vi "Compute Optimal IRF v4.vi"(6 "Laser Period":dbl[unit], 7 "Decay Fit Options":T1={"Show Fit Residuals"=TRUE, "Fit Model"=enum."1-Exponential", "Residual Type"=enum."Standard", "Max Decay Percentile"=0.0, "Min Decay Percentile"=0.0, "Show Full Decay"=TRUE, "Weights"=enum."Unweighted", "Fitting Method"=enum."Least Square", "Compute Parameter Uncertainties"=TRUE, "Periodic Boundaries"=TRUE, "Model Calculation"=enum."Simulation", "Period"=1.2500000000000001e-08, "Termination Criteria"={"Max Iterations"=0, "Max Function Calls"=0, "Max Time"=1000.0, "Function Tolerance"=1e-06, "Parameter Tolerance"=1e-06, "Gradient Tolerance"=0.0, "Min Lambda"=1e-06, "Max Lambda"=1e-06, "Initial Tick Count"=0}, "Offset Resolution"=1.2500000000000001e-08, "Use Local IRF"=TRUE, "Fitting Algorithm"=enum."Levenberg-Marquardt", "Show Confidence Interval "=TRUE, "Confidence Level"=95.0} {"Confidence Level" min=0.0 max=100.0; "Offset Resolution" min=0.0; "Period" min=0.0; "Min Decay Percentile" min=0.0 max=1.0; "Max Decay Percentile" min=0.0 max=100.0}, 8 "Error In":errorcluster, 9 "IRF Optimization Control":T12={"Search Range"=1e-18, "Search Step"=1e-18, "Tail Threshold (%)"=1e-09, "Regularized IRF"=FALSE, "Export Plot"=FALSE, "Export Data"=FALSE, "Smooth Metrics"=FALSE, "S-G Side Points"=1, "S-G Polynomial Order"=3, "Metrics"=enum."Tail Average"} {"S-G Polynomial Order" min=3 max=10; "S-G Side Points" min=1; "Tail Threshold (%)" min=0.0 max=100.0; "Search Range" min=0.0 max=1e-09}, 10 "Extract IRF Options":T8={"Time Constant for IRF Extraction"=1e-18, "IRF Order"=1, "Fourier Series Smoothing"=enum."None", "Noise Threshold"=0.0, "Smoothing Width"=0.0, "Fourier Series Truncation"=enum."Automatic", "Truncation Order"=0, "Save Power Spectrum"=FALSE, "Smoothing"=FALSE, "Smoothing Parameter"=0.0, "Smoothing Order"=1, "Method"=enum."Direct"} {"Smoothing Order" min=1 max=10; "Time Constant for IRF Extraction" format="%#_5g"}, 11 "Selected Plot Info":T14={"Multiplot XY Graph"=refnum, "Mouse Coordinates"={"Horizontal"=0, "Vertical"=0}, "Plot Index"=-1}) -> (0 "Error Out":errorcluster, 1 "Optimal Tau":dbl, 2 "Plot Name":string, 3 "IRF Plot":cluster{"X Array":dbl[], "Y Array":dbl[]}, 4 "Optimal IRF Results String":string, 5 "Optimization Graph":cluster{dbl[], dbl[]}[](graph))   [LabVIEW 2021, in "AlliGator IRF.lvlib"]
doc: "Extract IRF from provided decay and time constant"
uses:
  AlliGator/Decay Analysis/IRF/AlliGator IRF.lvlib
  Graphs/XY Graph/XY Graph Selected Plot Info.ctl
  Graphs/XY Graph/XY Graph Refnum.ctl
  <vilib>/Utility/miscctls.llb/LVPoint32TypeDef.ctl
  AlliGator/Decay Analysis/IRF/AlliGator IRF Optimization Controls.ctl
  AlliGator/Decay Analysis/IRF/AlliGator IRF Deconvolution Metrics.ctl
  IRF(X)PSED Extraction Options.ctl
  Fourier Series Smoothing Option.ctl
  Fourier Series Truncation.ctl
  IRF Extraction Method.ctl
  Decay Fit Options v4.ctl
  Decay Convolution/Decay Model.ctl
  Residual Type.ctl
  Fit Weights Type v2.ctl
  Non-linear Fitting Method v2.ctl
  Fit Calculation Method.ctl
  Non-linear Fitting Algorithm.ctl
  Fit Plot Request Information.ctl
  <vilib>/Utility/miscctls.llb/LVPointDoubleTypeDef.ctl
  Fit Models.ctl
  cc3fc4cb-3fe6-4f43-9f61-aa3a5ef9d036.vi
  <vilib>/Analysis/1siggen.llb/Ramp Pattern by Delta.vi
  Decay Convolution/LM model function and gradient (1-Exp, Convolved, Periodic, Fixed Parameters) v3.vi
  <userlib>/_OpenG.lib/array/array.llb/Filter 1D Array with Scalar (DBL)__ogtk.vi
  <userlib>/_OpenG.lib/array/array.llb/Delete Elements from 1D Array (DBL)__ogtk.vi
  <vilib>/Analysis/NI_AALBase.lvlib
  Time/Time.lvlib
  Fits.lvlib
  Utilities/Utilities.lvlib
  Arrays/Arrays.lvlib
  Graphs/XY Graph/XY Graph Add-Ons.lvlib
  <vilib>/Analysis/NI_AALPro.lvlib
  <userlib>/_OpenG.lib/array/array.llb/openg_array.lvlib
  AlliGator/Decay Analysis/Decay Fit/AlliGator Decay Fit.lvlib
panel:
  in  "Display":bool
  out "# Tail Points":i32
  out "min value":dbl
  in  "Debug":bool
  out "IRF Graph":cluster{"X Array":dbl[], "Y Array":dbl[]}[](graph)
  out "Current Tau (ns)":dbl format="%#_4g"
  # "1. In debug mode, move the cursor in the Optimization Graph to display the corresponding IRF in the IRF Graph\n2. Click on the close window X to stop debugging"
  # "see the AlliGator License on the block diagram (Ctrl+E or Window:Show Block Diagram)"
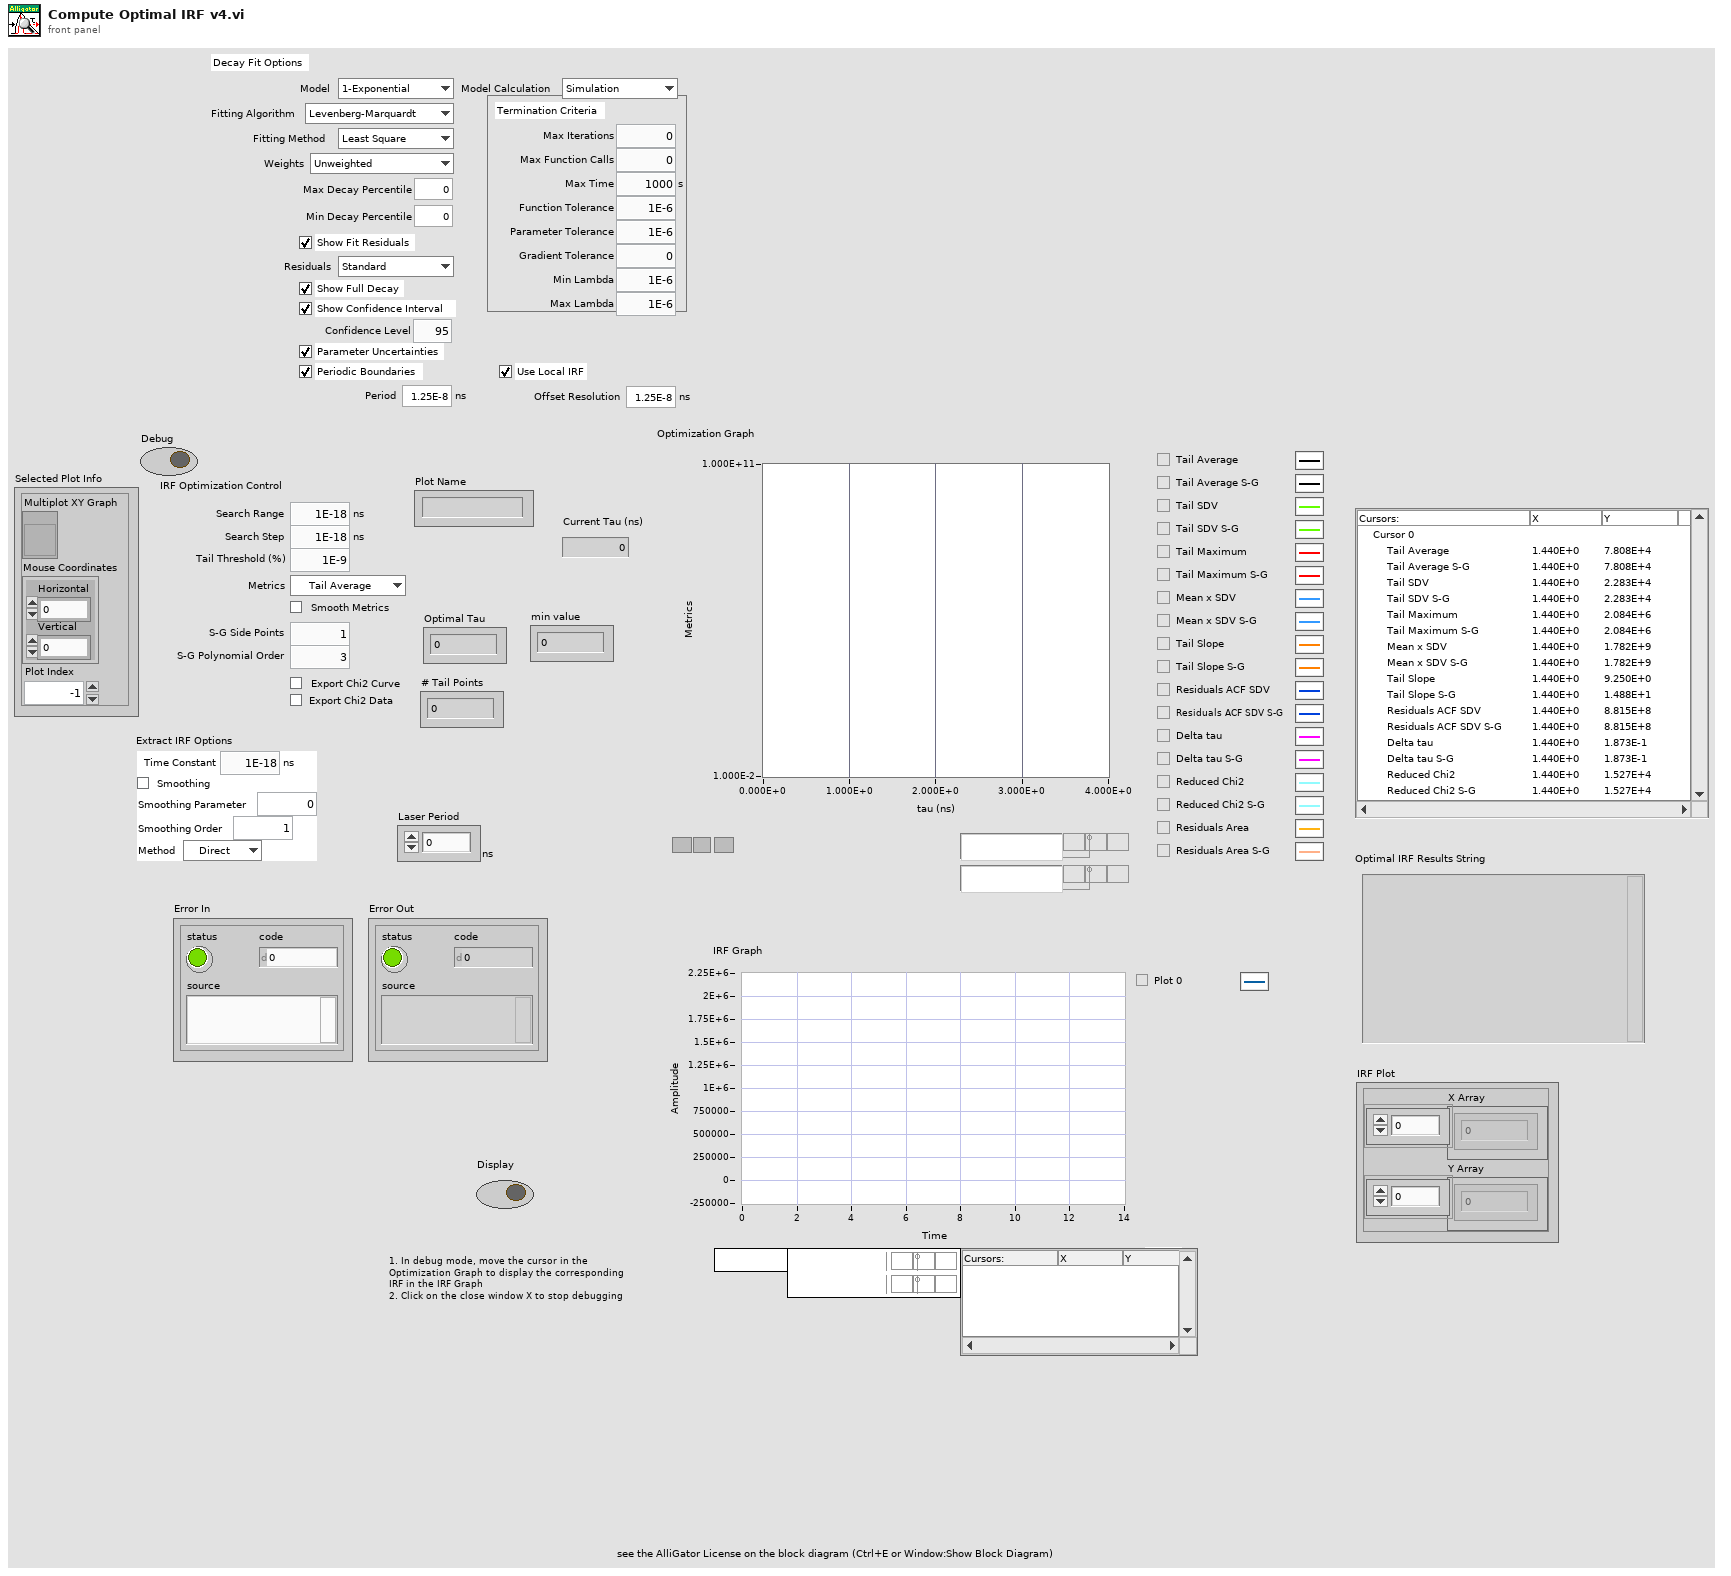
[diagram p1: front panel]
types:
  T1 = typedef "Fits.lvlib/Decay Fit Options v4.ctl" = cluster{"Show Fit Residuals":bool, "Fit Model":T2, "Residual Type":T3, "Max Decay Percentile":dbl, "Min Decay Percentile":dbl, "Show Full Decay":bool, "Weights":T4, "Fitting Method":T5, "Compute Parameter Uncertainties":bool, "Periodic Boundaries":bool, "Model Calculation":T6, "Period":dbl[unit], "Termination Criteria":cluster{"Max Iterations":i32, "Max Function Calls":i32, "Max Time":dbl[unit], "Function Tolerance":dbl, "Parameter Tolerance":dbl, "Gradient Tolerance":dbl, "Min Lambda":dbl, "Max Lambda":dbl, "Initial Tick Count":u32}, "Offset Resolution":dbl[unit], "Use Local IRF":bool, "Fitting Algorithm":T7, "Show Confidence Interval ":bool, "Confidence Level":dbl}
  T2 = typedef "Fits.lvlib/Decay Model.ctl" = enum16{"1-Exponential", "2-Exponentials"}
  T3 = typedef "Fits.lvlib/Residual Type.ctl" = enum16{"Standard", "Normalized", "Reduced"}
  T4 = typedef "Fits.lvlib/Fit Weights Type v2.ctl" = enum16{"Unweighted", "1/Variance (Neyman)", "1/Variance (Pearson)", "Best of All"}
  T5 = typedef "Fits.lvlib/Non-linear Fitting Method v2.ctl" = enum16{"Least Square", "Least Absolute Residual", "Bisquare", "MLE", "-", "Best of All"}
  T6 = typedef "Fits.lvlib/Fit Calculation Method.ctl" = enum16{"Simulation", "Convolution", "Integration"}
  T7 = typedef "Fits.lvlib/Non-linear Fitting Algorithm.ctl" = enum16{"Levenberg-Marquardt", "Trust-Region Dogleg"}
  T8 = typedef "Fits.lvlib/IRF(X)PSED Extraction Options.ctl" = cluster{"Time Constant for IRF Extraction":dbl[unit], "IRF Order":i32, "Fourier Series Smoothing":T9, "Noise Threshold":dbl, "Smoothing Width":dbl, "Fourier Series Truncation":T10, "Truncation Order":i32, "Save Power Spectrum":bool, "Smoothing":bool, "Smoothing Parameter":dbl, "Smoothing Order":u32, "Method":T11}
  T9 = typedef "Fits.lvlib/Fourier Series Smoothing Option.ctl" = enum16{"None", "Lanczos Factors", "Fejer Summation"}
  T10 = typedef "Fits.lvlib/Fourier Series Truncation.ctl" = enum16{"Automatic", "Fixed"}
  T11 = typedef "Fits.lvlib/IRF Extraction Method.ctl" = enum16{"Direct", "Topless", "Toeplitz"}
  T12 = typedef "AlliGator IRF.lvlib/AlliGator IRF Optimization Controls.ctl" = cluster{"Search Range":dbl[unit], "Search Step":dbl[unit], "Tail Threshold (%)":dbl, "Regularized IRF":bool, "Export Plot":bool, "Export Data":bool, "Smooth Metrics":bool, "S-G Side Points":i32, "S-G Polynomial Order":i32, "Metrics":T13}
  T13 = typedef "AlliGator IRF.lvlib/AlliGator IRF Deconvolution Metrics.ctl" = enum16{"Tail Average", "Tail SDV", "Tail Max", "Tail Average * SDV", "Tail Slope", "Residuals ACF SDV", "Delta tau", "Reduced Chi2", "Residuals Area"}
  T14 = typedef "XY Graph Add-Ons.lvlib/XY Graph Selected Plot Info.ctl" = cluster{"Multiplot XY Graph":T15, "Mouse Coordinates":T16, "Plot Index":i32}
  T15 = typedef "XY Graph Add-Ons.lvlib/XY Graph Refnum.ctl" = refnum<vi>
  T16 = typedef "LVPoint32TypeDef.ctl" = cluster{"Horizontal":i32, "Vertical":i32}
  T17 = typedef "Fits.lvlib/Fit Plot Request Information.ctl" = cluster{"XY Graph Ref":refnum<vi>, "Mouse Coordinates":T18, "Fit Model":T19, "Plot Index":i32}
  T18 = typedef "LVPointDoubleTypeDef.ctl" = cluster{"X":dbl, "Y":dbl}
  T19 = typedef "Fits.lvlib/Fit Models.ctl" = enum16{"Select a Fit Model...", "           Single Peak", "Gaussian", "Asymmetric Gaussian", "Lorentzian", "Asymmetric Lorentzian", "Gaussian/Lorentzian", "Lorentzian/Gaussian", "           Double Peak", "Two Gaussians", "Two Asymmetric Gaussians", "Two H-Connected Gaussians", "Two T-Connected Gaussians", "Two H-Connected Asymmetric Gaussians", "Two T-Connected Asymmetric Gaussians", "           Triple Peak", "Three Gaussians", "Three Asymmetric Gaussians", "              Decays", "1-Exponential", "IRF*PSED", "2-Exponentials", "            Power Law", "Power Law", "Power Law with Offset", "               ACF", "2D Gaussian ACF", "2D Gaussian + Blinking ACF", "2D Gaussian + Flow ACF", "3D Gaussian ACF", "3D Gaussian + Blinking ACF", "             Multiplot", "2D Gaussian ACF & 2D Gaussian + Flow ACF"}
  T20 = typedef "XY Graph Add-Ons.lvlib/XY Graph Plot Data.ctl" = cluster{"X Array":dbl[], "Y Array":dbl[]}
  T21 = typedef "Fits.lvlib/Decay Fit Parameter Constraints Arrays.ctl" = cluster{"Parameter Bounds (Fix+Fit)":cluster{"parameter minimum":dbl[], "parameter maximum":dbl[]}, "Fitted Parameters":T22[], "Fixed Parameters":T22[], "Fit Model":T2}
  T22 = typedef "Fits.lvlib/Decay Fit Parameters In List.ctl" = enum16{"Offset", "Baseline", "A_1", "tau_1", "A_2", "tau_2"}
  T23 = cluster{"t Array (dup)":dbl[], "IRF Array":dbl[]}
  T24 = typedef "Fits.lvlib/Fit Plots.ctl" = cluster{"Fitted Decay":cluster{"t Array":dbl[], "Fitted Array":dbl[]}, "Residuals":cluster{"t Array":dbl[], "Residual Array":dbl[]}, "Upper CI Plot":cluster{"t Array":dbl[], "Residual Array":dbl[]}, "Lower CI Plot":cluster{"t Array":dbl[], "Residual Array":dbl[]}}
  T25 = typedef "Fits.lvlib/Non-linear Fit Output v4.ctl" = cluster{"best nonlinear fit":dbl[], "best fit parameters":dbl[], "R^2":dbl, "RMSE":dbl, "error out":errorcluster, "Fitting Method":T26, "number of function calls":i32, "number of iterations":i32, "covariance":T27, "Chi 2":dbl, "DOF":i32, "Fit Convergence Criterion":T28, "Fitting Algorithm":T7, "Weighted Fit":T4, "Gradient":dbl, "|Delta Chi 2|":dbl, "|Delta Chi 2|/Chi 2":dbl, "Max |Delta a| /|a|":dbl, "Lambda":dbl, "RSS":dbl, "AIC":dbl, "BIC":dbl, "Max number of function calls":i32, "Max number of iterations":i32, "IRF":T20, "IRF Normalization Factor":dbl, "Decay Normalization Factor":dbl, "Number of offset fits":i32, "Weighted Chi2":dbl, "Unweighted Chi2":dbl}
  T26 = typedef "Fits.lvlib/Nonlinear Fit Method.ctl" = enum16{"Least Square", "Least Absolute Residual", "Bisquare", "MLE"}
  T27 = typedef "NI_Matrix.lvlib/RealMatrix.ctl" = dbl[][]
  T28 = typedef "Fits.lvlib/Convergence Criteria.ctl" = enum16{"Continue", "Tolerances Exceeded", "Max Time Exceeded", "Max Iterations Exceeded", "Max Function Evaluations Exceeded", "Scale Range Exceeded"}
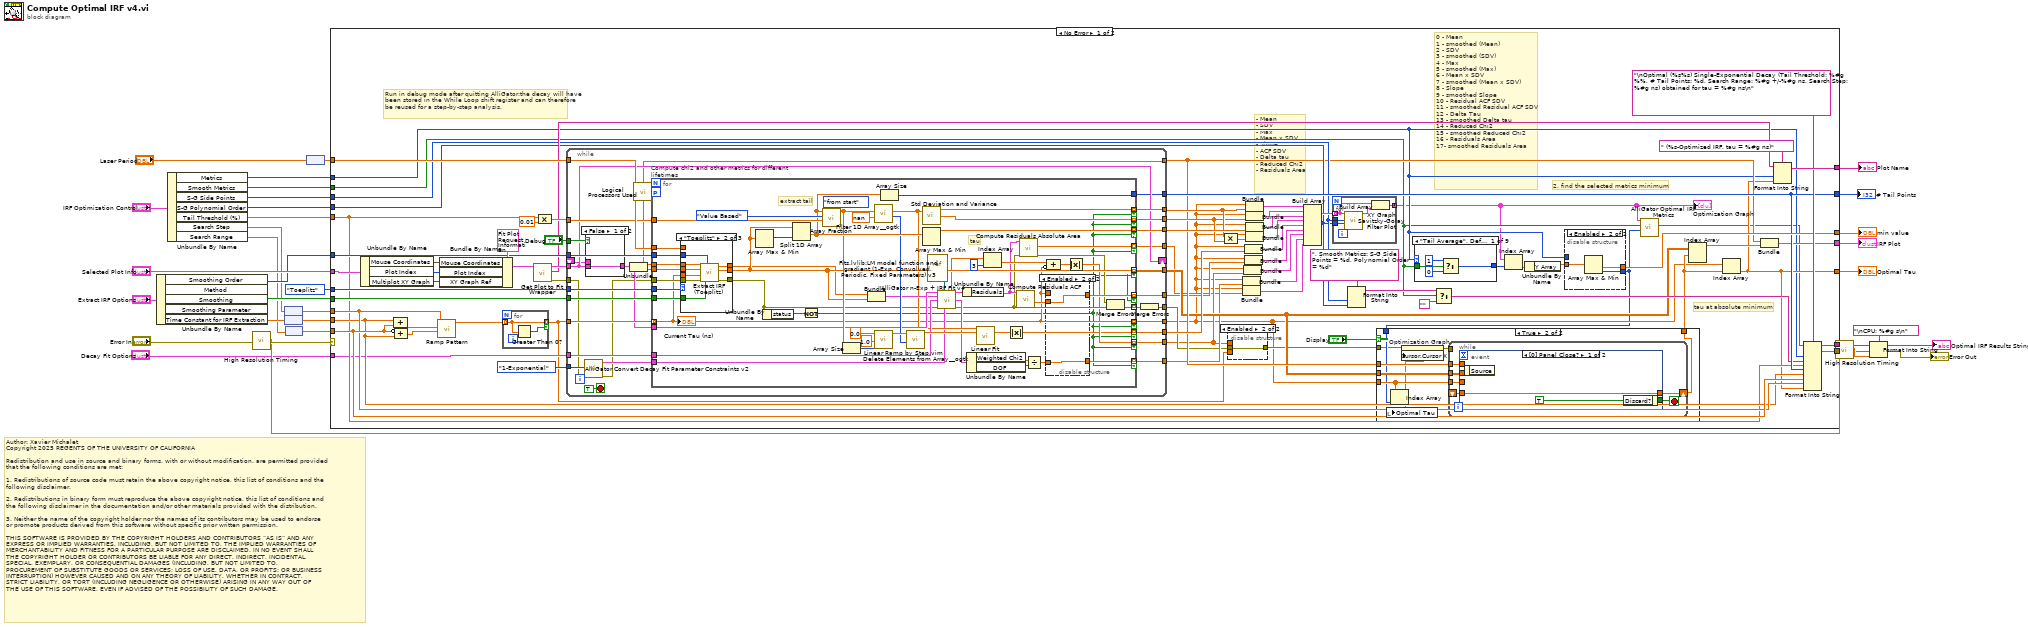
[diagram p0: block diagram]
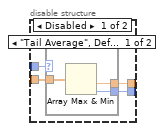
[diagram p2: hidden frame]
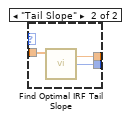
[diagram p3: hidden frame]
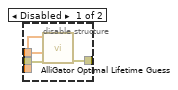
[diagram p4: hidden frame]
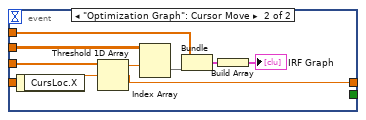
[diagram p6: hidden frame]
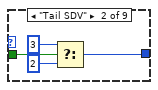
[diagram p7: hidden frame]
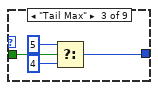
[diagram p8: hidden frame]
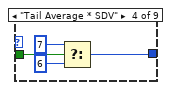
[diagram p9: hidden frame]
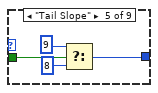
[diagram p10: hidden frame]
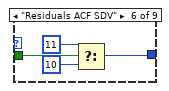
[diagram p11: hidden frame]
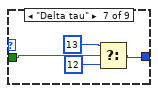
[diagram p12: hidden frame]
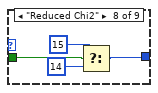
[diagram p13: hidden frame]
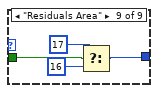
[diagram p14: hidden frame]
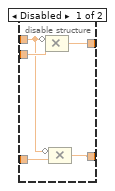
[diagram p15: hidden frame]
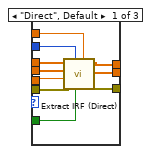
[diagram p16: hidden frame]
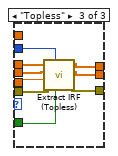
[diagram p17: hidden frame]
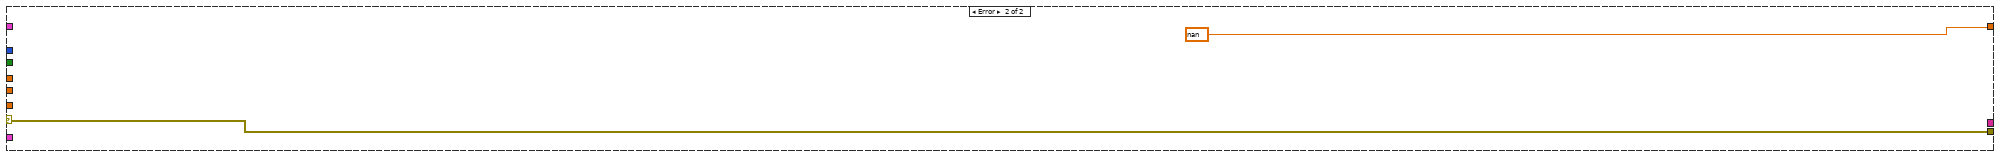
[diagram p19: hidden frame]
diagram:
  # "Author: Xavier Michalet\nCopyright 2025 REGENTS OF THE UNIVERSITY OF CALIFORNIA\n\nRedistribution and use in source and binary forms, with or without modification, are permitted provided\nthat the following conditions are met:\n\n1. Redistributions of source code must retain the above copyright notice, this list of conditions and the\nfollowing disclaimer.\n\n2. Redistributions in binary form must reproduce the above copyright notice, this list of conditions and\nthe following disclaimer in the documentation and/or other materials provided with the distribution.\n\n3. Neither the name of the copyright holder nor the names of its contributors may be used to endorse \nor promote products derived from this software without specific prior written permission.\n\nTHIS SOFTWARE IS PROVIDED BY THE COPYRIGHT HOLDERS AND CONTRIBUTORS “AS IS” AND ANY \nEXPRESS OR IMPLIED WARRANTIES, INCLUDING, BUT NOT LIMITED TO, THE IMPLIED WARRANTIES OF\nMERCHANTABILITY AND FITNESS FOR A PARTICULAR PURPOSE ARE DISCLAIMED. IN NO EVENT SHALL\nTHE COPYRIGHT HOLDER OR CONTRIBUTORS BE LIABLE FOR ANY DIRECT, INDIRECT, INCIDENTAL, \nSPECIAL, EXEMPLARY, OR CONSEQUENTIAL DAMAGES (INCLUDING, BUT NOT LIMITED TO, \nPROCUREMENT OF SUBSTITUTE GOODS OR SERVICES; LOSS OF USE, DATA, OR PROFITS; OR BUSINESS\nINTERRUPTION) HOWEVER CAUSED AND ON ANY THEORY OF LIABILITY, WHETHER IN CONTRACT, \nSTRICT LIABILITY, OR TORT (INCLUDING NEGLIGENCE OR OTHERWISE) ARISING IN ANY WAY OUT OF\nTHE USE OF THIS SOFTWARE, EVEN IF ADVISED OF THE POSSIBILITY OF SUCH DAMAGE."
  n1 = Unbundle By Name("Extract IRF Options") -> ("Smoothing Order"=w21:u32, "Smoothing"=w20:bool, "Time Constant for IRF Extraction"=w23:dbl[unit])  [unwired: 2 out]
  n2 = Unbundle By Name("IRF Optimization Control") -> ("Metrics"=w5:T13, "Smooth Metrics"=w8:bool, "S-G Side Points"=w7:i32, "S-G Polynomial Order"=w6:i32, "Tail Threshold (%)"=w15:dbl, "Search Step"=w14:dbl[unit], "Search Range"=w12:dbl[unit])
  n3 = call "High Resolution Timing.vi"("Error In"="Error In") -> ("elapsed (relative) seconds"=w30:dbl, "Error Out"=w34:errorcluster)  [unwired: 16 in, 1 out]
  n4 = node(w14) -> (w33:dbl)
  n5 = node(w23) -> (w32:dbl)
  n6 = node(w12) -> (w11:dbl)
  n7 = node("Laser Period") -> (w17:dbl)
  n8 = case shown="No Error" w34 {
    selector: w34 -> [_ w325]
    tunnel: [w94 w325] -> w35
    tunnel: w32 -> [w76 _]
    tunnel: w33 -> [w81 _]
    tunnel: w11 -> [w82 _]
    tunnel: "Selected Plot Info" -> [w109 _]
    tunnel: [w95 _] -> w29
    tunnel: [w62 _] -> w22
    tunnel: w21 -> [w102 _]
    tunnel: w20 -> [w101 _]
    tunnel: [w50 nan] -> w19
    tunnel: [w97 _] -> w18
    tunnel: w15 -> [w71 _]
    tunnel: IRF_Extraction_Method."Toeplitz" ("Method") -> [w93 _]
    tunnel: w17 -> [w92 _]
    tunnel: [w79 _] -> w10
    tunnel: [w77 _] -> w9
    tunnel: w8 -> [w39 _]
    tunnel: w7 -> [w68 _]
    tunnel: w6 -> [w67 _]
    tunnel: w5 -> [w49 _]
    tunnel: "Decay Fit Options" -> [w56 _]
    frame No Error {
      # "Run in debug mode after quitting AlliGator:the decay will have been stored in the While Loop shift register and can therefore be reused for a step-by-step analysis."
      # "0 - Mean\n1 - smoothed (Mean)\n2 - SDV\n3 - smoothed (SDV)\n4 - Max\n5 - smoothed (Max)\n6 - Mean x SDV\n7 - smoothed (Mean x SDV)\n8 - Slope\n9 - smoothed Slope\n10 - Residual ACF SDV\n11 - smoothed Residual ACF SDV\n12 - Delta Tau\n13 - smoothed Delta tau\n14 - Reduced Chi2\n15 - smoothed Reduced Chi2\n16 - Residuals Area\n17- smoothed Residuals Area"
      # "- Mean\n- SDV\n- Max\n- Mean x SDV\n- Slope\n- ACF SDV\n- Delta tau\n- Reduced Chi2\n- Residuals Area"
      # "tau at absolute minimum"
      # "2. find the selected metrics minimum"
      n9 = Unbundle By Name(w109) -> ("Mouse Coordinates"=w106:T16, "Plot Index"=w105:i32, "Multiplot XY Graph"=w107:T15)
      n10 = Compound Arithmetic op=ADD(w76, w82) -> (w111:dbl)
      n11 = Compound Arithmetic op=ADD(invert w82, w76) -> (w110:dbl)
      n12 = call-poly <vilib>:"Ramp Pattern.vi"("start"=w110, "end"=w111, "delta"=w81) -> ("Ramp Pattern"=w80:dbl[])  [unwired: 6 in, 2 out]
      n13 = Bundle By Name(cluster=T17 {"XY Graph Ref"=refnum, "Mouse Coordinates"={"X"=0.0, "Y"=0.0}, "Fit Model"=enum."IRF*PSED", "Plot Index"=-1} ("Fit Plot Information"), "Mouse Coordinates"=w106, "Plot Index"=w105, "XY Graph Ref"=w107) -> (w103:T17)
      n14 = for {
        tunnel: w80 -> [w192] mode=indexing
        tunnel: [w192] -> w44 mode=indexing if=w191
        n15 = Greater Than 0?(x=w192) -> (x > 0?=w191:bool)
      }
      n16 = call "Get Plot to Fit Wrapper.vi"("Fit Plot Information"=w103) -> ("error out"=w91:errorcluster, "Plot Name"=w75:string, "Clipped Plot"=w104:T20)  [unwired: 4 in, 4 out]
      n17 = Compound Arithmetic op=MULTIPLY(w71, 0.01 ("value")) -> (w89:dbl)
      n18 = while {
        tunnel: w104 -> [w209]
        tunnel: [w223] -> w57
        tunnel: w102 -> [w222]
        tunnel: w101 -> [w221]
        tunnel: w44 -> [w220]
        tunnel: w93 -> [w219]
        tunnel: w92 -> [w218]
        tunnel: w91 -> [w195]
        tunnel: w89 -> [w217]
        tunnel: [w216] -> w87
        tunnel: [w215] -> w41
        tunnel: [w214] -> w85
        tunnel: [w213] -> w78
        tunnel: "Debug" -> [w211]
        shift-right: [w209] -> _
        shift-left: _ -> [w208]
        tunnel: [w207] -> w77
        tunnel: [w206] -> w58
        tunnel: [w205] -> w60
        tunnel: w56 -> [w203]
        tunnel: [w201] -> w46
        tunnel: [w200] -> w55
        tunnel: [w199] -> w43
        tunnel: Decay_Model."1-Exponential" ("Fit Model") -> [w197]
        tunnel: [w194] -> w48
        tunnel: [w193] -> w42
        stop <- TRUE stop-if-true
        n19 = call "AlliGator Convert Decay Fit Parameter Constraints v2.vi"("Error In"=w195, "Fit Model"=w197) -> ("Error Out"=w196:errorcluster, "All Parameter Constraints"=w198:T21)  [unwired: 7 in, 1 out]
        n20 = case shown="False" w211 {
          tunnel: w209 -> [w317 _]
          tunnel: [w317 w318] -> w204
          tunnel: w208 -> [_ w318]
          frame False {
          }
          frame True {
          }
        }
        n21 = Unbundle(w204) -> ("X Array"=w206:dbl[], "Y Array"=w210:dbl[])
        n22 = call "Logical Processors Used.vi"() -> ("# Logical Processor Used"=w224:i32)  [unwired: 6 in]
        n23 = for "Compute chi2 and other metrics for different lifetimes" {
          tunnel: w220 -> [w234] mode=indexing
          workers-P: w224 -> [_]
          tunnel: w206 -> [w279]
          tunnel: w210 -> [w281]
          tunnel: w196 -> [w280]
          tunnel: [w254] -> w223 mode=indexing if=w225
          tunnel: w222 -> [w278]
          tunnel: w221 -> [w277]
          tunnel: [w276] -> w213 mode=indexing if=w225
          tunnel: [w234] -> w215 mode=indexing if=w225
          tunnel: w217 -> [w271]
          tunnel: w219 -> [w274]
          tunnel: w218 -> [w242]
          tunnel: [w273] -> w214 mode=indexing if=w225
          tunnel: [w266] -> w216 mode=indexing if=w225
          tunnel: [w270] -> w207
          tunnel: [w231] -> w205 mode=indexing if=w225
          tunnel: w204 -> [w255]
          tunnel: w203 -> [w251]
          tunnel: [w228] -> w202 mode=indexing
          tunnel: [w237] -> w200 mode=indexing if=w225
          tunnel: [w232] -> w199 mode=indexing if=w225
          tunnel: w198 -> [w241]
          tunnel: [w235] -> w194 mode=indexing if=w225
          tunnel: [w226] -> w193 mode=indexing if=w225
          # "tau"
          # "extract tail"
          n24 = case shown="\"Toeplitz\"" w274 {
            tunnel: w281 -> [w297 w307 w315]
            tunnel: w280 -> [w295 w306 w314]
            tunnel: w279 -> [w298 w305 w316]
            tunnel: w278 -> [w292 w304 w309]
            tunnel: w277 -> [w291 w303 w310]
            tunnel: [w293 w302 w312] -> w254
            tunnel: [w294 w301 w311] -> w249
            tunnel: w234 -> [w296 w300 w313]
            tunnel: w242 -> [w290 _ _]
            tunnel: [w289 w299 w308] -> w252
            frame "Direct", Default {
              n25 = call "Extract IRF (Direct).vi"("Period"=w290, "Tail Smoothing (T)"=w291, "Smoothing Order"=w292, "Error In"=w295, "Time Constant"=w296, "Intensity Array"=w297, "t Array"=w298) -> ("Error Out"=w294:errorcluster, "IRF Array"=w293:dbl[], "t Array (dup)"=w289:dbl[])  [unwired: 1 in, 1 out]
            }
            frame "Toeplitz" {
              n26 = call "Extract IRF (Toeplitz).vi"("Tail Smoothing (T)"=w303, "Smoothing Order"=w304, "Error In"=w306, "Time Constant"=w300, "Intensity Array"=w307, "t Array"=w305) -> ("Error Out"=w301:errorcluster, "IRF Array"=w302:dbl[], "t Array (dup)"=w299:dbl[])  [unwired: 2 in, 1 out]
            }
            frame "Topless" {
              n27 = call "Extract IRF (Topless).vi"("Tail Smoothing (T)"=w310, "Smoothing Order"=w309, "Error In"=w314, "Time Constant"=w313, "Intensity Array"=w315, "t Array"=w316) -> ("Error Out"=w311:errorcluster, "IRF Array"=w312:dbl[], "t Array (dup)"=w308:dbl[])  [unwired: 2 in, 1 out]
            }
          }
          n28 = Array Max & Min(array=w254) -> (max index (indices)=w272:i32)  [unwired: 3 out]
          n29 = Unbundle By Name(w249) -> ("status"=w275:bool)
          n30 = Split 1D Array(array=w254, index=w272) -> (second subarray=w267:dbl[])  [unwired: 1 out]
          n31 = Not(x=w275) -> (.not. x?=w225:bool)
          n32 = call "Array Fraction.vi"("Direction (from start)"=enum16{"from start", "from end"}."from start", "fraction [0, 1]"=w271, "Method (Length Based)"=enum16{"Value Based", "Length Based"}."Value Based", "Array"=w267) -> ("Array out"=w261:dbl[])  [unwired: 6 in, 1 out]
          n33 = Array Size(array=w261) -> (size(s)=w260:i32)
          n34 = Bundle("t Array (dup)"=w252, "IRF Array"=w254) -> (w253:T23)  [unwired: 1 in]
          n35 = call-poly <userlib>:"Filter 1D Array__ogtk.vi"("items to filter"=nan, "array"=w261) -> ("filtered item indices"=w257:i32[], "filtered array"=w250:dbl[])  [unwired: 4 in]
          n36 = call "Linear Ramp by Step.vim"("# Elements (1)"=w260, "Step (1)"=1.0, "Start (0)"=0.0) -> ("Ramp"=w259:dbl[])  [unwired: 8 in]
          n37 = Array Size(array=w267) -> (size(s)=w270:i32)
          n38 = call-poly <userlib>:"Delete Elements from Array__ogtk.vi"("indices"=w257, "array"=w259) -> ("array w/ subset deleted"=w258:dbl[])  [unwired: 8 in, 1 out]
          n39 = call <vilib>:"Std Deviation and Variance.vi"("X"=w250) -> ("mean"=w273:dbl, "standard deviation"=w276:dbl)  [unwired: 1 in, 1 out]
          n40 = Array Max & Min(array=w267) -> (max value=w266:dbl)  [unwired: 3 out]
          n41 = vi-ref "Fits.lvlib:LM model function and gradient (1-Exp, Convolved, Periodic, Fixed Parameters) v3.vi"() -> (w256:refnum<vi>)
          n42 = call "AlliGator n-Exp + IRF Fit v4.vi"("Decay"=w255, "VI Refnum"=w256, "IRF"=w253, "Fit Options"=w251, "error in (no error)"=w249, "All Parameter Constraints"=w241) -> ("All unscaled Fit Parameters (w tau)"=w245:dbl[], "Fit Plots"=w247:T24, "Fit Output"=w240:T25, "error out"=w229:errorcluster)  [unwired: 2 in, 4 out]
          n43 = Unbundle By Name(w247) -> ("Residuals"=w230:cluster{"t Array":dbl[], "Residual Array":dbl[]})
          n44 = Unbundle By Name(w240) -> ("Weighted Chi2"=w239:dbl, "DOF"=w238:i32)
          n45 = call <vilib>:"Linear Fit.vi"("Y"=w250, "X"=w258) -> ("slope"=w265:dbl)  [unwired: 9 in, 4 out]
          n46 = Index Array(array=w245, index=3) -> (element=w243:dbl)
          n47 = Absolute Value(x=w265) -> (abs(x)=w231:dbl)
          n48 = call "Compute Residuals ACF.vi"("Error In"=w229, "Residual Plot in"=w230) -> ("Error Out"=w248:errorcluster, "ACF SDV"=w246:dbl)  [unwired: 5 in, 3 out]
          n49 = call "Compute Residuals Absolute Area.vi"("Error In"=w229, "Residual Plot in"=w230) -> ("Error Out"=w227:errorcluster, "Residuals Area"=w226:dbl)  [unwired: 7 in, 1 out]
          n50 = Divide(x=w239, y=w238) -> (x/y=w236:dbl)
          n51 = disable-structure shown="Enabled" {
            disable-tunnel: w246 -> [w286 w287]
            disable-tunnel: [w285 w287] -> w237
            disable-tunnel: w236 -> [w284 w288]
            disable-tunnel: [w283 w288] -> w235
            disable-tunnel: w234 -> [w282 _]
            frame Disabled {
              n52 = Compound Arithmetic op=MULTIPLY(invert w282, w286) -> (w285:dbl)
              n53 = Compound Arithmetic op=MULTIPLY(invert w282, w284) -> (w283:dbl)
            }
            frame Enabled {
            }
          }
          n54 = Compound Arithmetic op=ADD(w243, invert w234) -> (w233:dbl)
          n55 = Absolute Value(x=w233) -> (abs(x)=w232:dbl)
          n56 = Merge Errors(w227, w248) -> (w228:errorcluster)
          "Current Tau (ns)" <- w234
        }
        n57 = Merge Errors(w202) -> (w201:errorcluster)
      }
      n58 = Compound Arithmetic op=MULTIPLY(w85, w78) -> (w84:dbl[])
      n59 = disable-structure shown="Enabled" {
        disable-tunnel: w46 -> [w128 w129]
        disable-tunnel: [w127 w129] -> w45
        disable-tunnel: w44 -> [w126 _]
        disable-tunnel: w43 -> [w125 _]
        frame Disabled {
          n60 = call "AlliGator Optimal Lifetime Guess.vi"("error in (no error)"=w128, "Delta tau Array"=w125, "Guessed tau Array"=w126) -> ("error out"=w127:errorcluster)  [unwired: 7 in, 1 out]
        }
        frame Enabled {
        }
      }
      n61 = Bundle(w41, w48) -> (w47:cluster{dbl[], dbl[]})  [unwired: 1 in]
      n62 = Bundle(w41, w42) -> (w40:cluster{dbl[], dbl[]})  [unwired: 1 in]
      n63 = Bundle(w41, w43) -> (w52:cluster{dbl[], dbl[]})  [unwired: 1 in]
      n64 = Bundle(w41, w60) -> (w53:cluster{dbl[], dbl[]})  [unwired: 1 in]
      n65 = Bundle(w41, w55) -> (w54:cluster{dbl[], dbl[]})  [unwired: 1 in]
      n66 = Bundle(w41, w85) -> (w100:cluster{dbl[], dbl[]})  [unwired: 1 in]
      n67 = Bundle(w41, w78) -> (w99:cluster{dbl[], dbl[]})  [unwired: 1 in]
      n68 = Bundle(w41, w87) -> (w90:cluster{dbl[], dbl[]})  [unwired: 1 in]
      n69 = Bundle(w41, w84) -> (w86:cluster{dbl[], dbl[]})  [unwired: 1 in]
      n70 = Build Array(w100, w99, w90, w86, w53, w54, w52, w47, w40) -> (w74:cluster{dbl[], dbl[]}[])
      n71 = for {
        tunnel: w74 -> [w321] mode=indexing
        tunnel: [w322] -> w38 mode=concatenating
        tunnel: w68 -> [w320]
        tunnel: w67 -> [w319]
        n72 = call "XY Graph Savitzky-Golay Filter Plot.vi"("polynomial order  (3)"=w319, "side points (6)"=w320, "Plot in"=w321) -> ("Plot out"=w323:cluster{"X Array":dbl[], "Y Array":dbl[]})  [unwired: 7 in, 1 out]
        n73 = Build Array(w321, w323) -> (w322:cluster{"X Array":dbl[], "Y Array":dbl[]}[])
      }
      "Optimization Graph" <- w38
      n74 = Format Into String(format string=", Smooth Metrics: S-G Side Points = %d, Polynomial Order = %d" ("initial string"), w68, w67) -> (resulting string=w69:string)  [unwired: 2 in, 1 out]
      n75 = case shown="\"Tail Average\", Default" w49 {
        tunnel: w39 -> [w158 w162 w166 w170 w173 w177 w182 w185 w189]
        tunnel: [w155 w159 w163 w167 w171 w175 w179 w183 w187] -> w64
        frame "Tail Average", Default {
          n76 = Select(t=1, s=w158, f=0) -> (s? t:f=w155:i32)
        }
        frame "Tail SDV" {
          n77 = Select(t=3, s=w162, f=2) -> (s? t:f=w159:i32)
        }
        frame "Tail Max" {
          n78 = Select(t=5, s=w166, f=4) -> (s? t:f=w163:i32)
        }
        frame "Tail Average * SDV" {
          n79 = Select(t=7, s=w170, f=6) -> (s? t:f=w167:i32)
        }
        frame "Tail Slope" {
          n80 = Select(t=9 ("f"), s=w173, f=8) -> (s? t:f=w171:i32)
        }
        frame "Residuals ACF SDV" {
          n81 = Select(t=11 ("f"), s=w177, f=10) -> (s? t:f=w175:i32)
        }
        frame "Delta tau" {
          n82 = Select(t=13 ("f"), s=w182, f=12) -> (s? t:f=w179:i32)
        }
        frame "Reduced Chi2" {
          n83 = Select(t=15 ("f"), s=w185, f=14) -> (s? t:f=w183:i32)
        }
        frame "Residuals Area" {
          n84 = Select(t=17 ("f"), s=w189, f=16) -> (s? t:f=w187:i32)
        }
      }
      n85 = Select(t=w69, s=w39, f="") -> (s? t:f=w65:string)
      n86 = Index Array(array=w38, index=w64) -> (element=w73:cluster{"X Array":dbl[], "Y Array":dbl[]})
      n87 = Unbundle By Name(w73) -> ("Y Array"=w72:dbl[])
      n88 = disable-structure shown="Enabled" {
        disable-tunnel: [w115 w124] -> w79
        disable-tunnel: w72 -> [w114 w123]
        disable-tunnel: [w113 w122] -> w37
        disable-tunnel: w49 -> [w112 _]
        frame Disabled {
          n89 = case shown="\"Tail Average\", Default" w112 {
            tunnel: [w118 w120] -> w115
            tunnel: w114 -> [w117 w121]
            tunnel: [w116 w119] -> w113
            frame "Tail Average", Default {
              n90 = Array Max & Min(array=w117) -> (min value=w118:dbl, min index (indices)=w116:i32)  [unwired: 2 out]
            }
            frame "Tail Slope" {
              n91 = call "Find Optimal IRF Tail Slope.vi"("Slope Array"=w121) -> ("Optimal Index"=w119:i32, "Optimal Slope"=w120:dbl)  [unwired: 9 in]
            }
          }
        }
        frame Enabled {
          n92 = Array Max & Min(array=w123) -> (min value=w124:dbl, min index (indices)=w122:i32)  [unwired: 2 out]
        }
      }
      n93 = case shown="True" "Display" {
        tunnel: w41 -> [_ w134]
        tunnel: w57 -> [_ w138]
        tunnel: w37 -> [w130 w133]
        tunnel: [w130 w136] -> w59
        tunnel: w58 -> [_ w137]
        tunnel: w45 -> [_ w131]
        frame False {
        }
        frame True {
          n94 = Index Array(array=w134, index=w133) -> (element=w132:dbl)
          n95 = local write "Optimal Tau"(w132) -> ()
          n96 = property on="Optimization Graph" class="XYGraph (strict)"(error in=w131, "Cursor.Cursor X"=w132) -> (error out=w135:errorcluster)  [unwired: 1 in, 1 out]
          n97 = while {
            tunnel: w134 -> [w143]
            tunnel: w138 -> [w142]
            tunnel: w137 -> [w141]
            shift-right: [w140] -> w136
            shift-left: _ -> [w139]
            tunnel: w135 -> [_]
            stop <- w144 stop-if-true
            n98 = event shown="[0] Panel Close?" {
              selector: _ -> [_ _]
              dyn-events: _ -> [_ _]
              timeout: _ -> [_ _]
              tunnel: [w146 _] -> w144
              tunnel: w143 -> [_ w151]
              tunnel: w142 -> [_ w153]
              tunnel: w141 -> [_ w148]
              tunnel: [w145 w147] -> w140
              tunnel: w139 -> [w145 _]
              event Panel Close? {
                w146 = TRUE ("Discard?")
                n99 = event-data() -> ()  [unwired: 1 in, 1 out]
                n100 = event-data("Discard?"=w146) -> ()  [unwired: 1 in, 1 out]
              }
              event "Optimization Graph": Cursor Move {
                n101 = event-data() -> ("CursLoc.X"=w154:dbl)  [unwired: 1 in]
                n102 = Threshold 1D Array(2:w154, 3:w151) -> (0:w147:dbl)  [unwired: 1 in]
                n103 = Index Array(array=w153, index (row)=w147) -> (element=w152:dbl[])  [unwired: 1 in]
                n104 = Bundle("X Array"=w148, "IRF Array"=w152) -> (w150:cluster{"X Array":dbl[], "IRF Array":dbl[]})  [unwired: 1 in]
                n105 = Build Array(w150) -> (→"IRF Graph":cluster{"X Array":dbl[], "IRF Array":dbl[]}[])
              }
            }
          }
        }
      }
      n106 = call "AlliGator Optimal IRF Metrics.vi"("index"=w37, "Smooth Metrics"=w39, "Plot Array"=w38) -> ("Message"=w36:string)  [unwired: 7 in, 1 out]
      n107 = Index Array(array=w57, index (row)=w59) -> (element=w63:dbl[])  [unwired: 1 in]
      n108 = Index Array(array=w41, index=w59) -> (element=w50:dbl)
      n109 = Bundle("X Array"=w58, "IRF Array"=w63) -> (w62:cluster{"X Array":dbl[], "IRF Array":dbl[]})  [unwired: 1 in]
      n110 = Format Into String(format string=" (%s-Optimized IRF, tau = %#g ns)", initial string=w75, w49, w50) -> (resulting string=w97:string)  [unwired: 1 in, 1 out]
      n111 = Format Into String(format string="\nOptimal (%s%s) Single-Exponential Decay (Tail Threshold: %#g %%, # Tail Points: %d, Search Range: %#g +/-%#g ns, Search Step: %#g ns) obtained for tau = %#g ns\n" ("string"), initial string=w36, w49, w65, w71, w77, w76, w82, w81, w50) -> (resulting string=w95:string, error out=w94:errorcluster)  [unwired: 1 in]
    }
    frame Error {
    }
  }
  "Optimal Tau" <- w19
  "Plot Name" <- w18
  "IRF Plot" <- w22
  "min value" <- w10
  "# Tail Points" <- w9
  n112 = call "High Resolution Timing.vi"("relative seconds (NaN)"=w30, "Error In"=w35) -> ("elapsed (relative) seconds"=w27:dbl, "Error Out"=w25:errorcluster)  [unwired: 15 in, 1 out]
  n113 = Format Into String(format string="\nCPU: %#g s\n", initial string=w29, error in=w25, w27) -> (resulting string=→"Optimal IRF Results String":string, error out=→"Error Out":errorcluster)
